vi "PID Control.vi"(8 "Reset Encoder 0":bool, 9 "M2 Setpoint":dbl(slide) scale=-0.5..0.5, 10 "M1 Setpoint":dbl(slide) scale=-0.5..0.5, 11 "M0 Setpoint":dbl(slide) scale=-1.0..1.0) -> (2 "Speed Cluster":T1, 3 "Distance Cluster":T2)   [LabVIEW 2018]
uses:
  <vilib>/addons/control/pid/pid.llb/PID (DBL).vi
  <vilib>/addons/control/pid/NI_PID_pid.lvlib
panel:
  out "dt out (s)":dbl format="%.3f"
  in  "stop":bool
  out "PID tuning Chart":dynamicdata(graph)
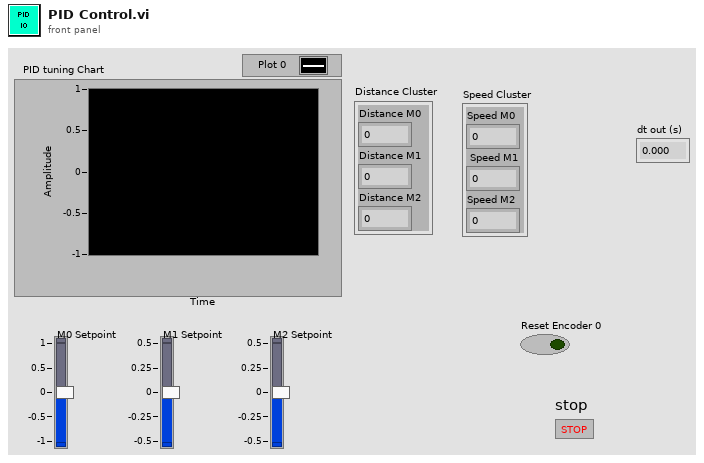
[diagram p1: front panel]
types:
  T1 = cluster{"Speed M0":dbl, " Speed M1":dbl, "Speed M2":dbl}
  T2 = cluster{"Distance M0 ":dbl, "Distance M1 ":dbl, "Distance M2 ":dbl}
  T3 = cluster{"proportional gain (Kc)":dbl, "integral time (Ti, min)":dbl, "derivative time (Td, min)":dbl}
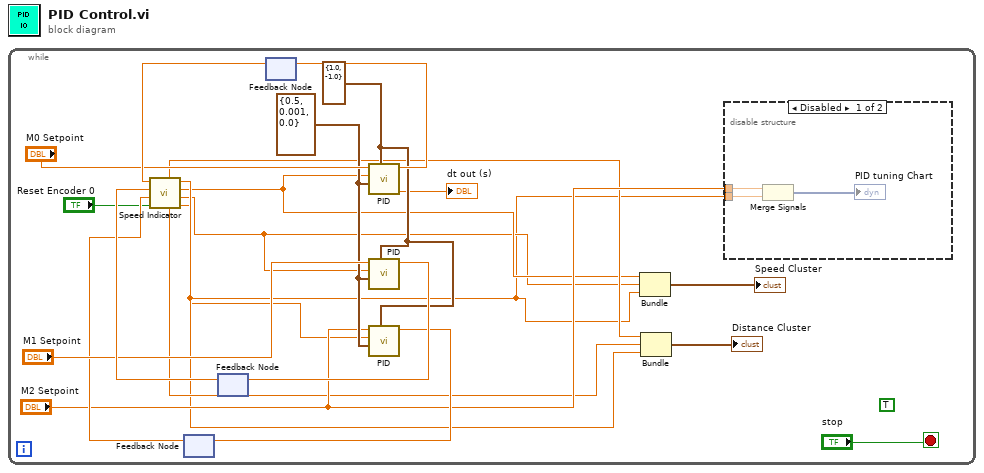
[diagram p0: block diagram]
diagram:
  n1 = while {
    stop <- "stop" stop-if-true
    (unwired) TRUE ("Boolean")
    w16 = T3 {"proportional gain (Kc)"=0.5, "integral time (Ti, min)"=0.001, "derivative time (Td, min)"=0.0} ("PID gains")
    w13 = cluster{"output high":dbl, "output low":dbl} {"output high"=1.0, "output low"=-1.0} ("output range")
    n2 = feedback #1() -> (w14:dbl)  [unwired: 1 in]
    n3 = feedback #2() -> (w18:dbl)  [unwired: 1 in]
    n4 = feedback #3() -> (w22:dbl)  [unwired: 1 in]
    n5 = call "Speed Indicator.vi"("Reset Encoder 0"="Reset Encoder 0", "Speed M2"=w14, "Speed M1 2"=w18, "Speed M0"=w22) -> ("Speed M2"=w5:dbl, "Speed M1"=w6:dbl, "Speed M0"=w7:dbl, "Distance M2"=w9:dbl, "Distance M1"=w10:dbl, "Distance M0"=w11:dbl)  [unwired: 2 in]
    n6 = call-poly <vilib>:"PID.vi"("output range"=w13, "PID gains"=w16, "process variable"=w7, "setpoint"="M0 Setpoint") -> ("dt out (s)"=→"dt out (s)":dbl, "output"=w21:dbl)  [unwired: 6 in]
    n7 = feedback-in #3(w21) -> ()
    n8 = call-poly <vilib>:"PID.vi"("output range"=w13, "PID gains"=w16, "process variable"=w6, "setpoint"="M1 Setpoint") -> ("output"=w19:dbl)  [unwired: 6 in, 1 out]
    n9 = feedback-in #2(w19) -> ()
    n10 = call-poly <vilib>:"PID.vi"("output range"=w13, "PID gains"=w16, "process variable"=w5, "setpoint"="M2 Setpoint") -> ("output"=w15:dbl)  [unwired: 6 in, 1 out]
    n11 = feedback-in #1(w15) -> ()
    n12 = Bundle("Speed M0"=w7, "Speed M1"=w6, "Speed M2"=w5) -> (→"Speed Cluster":T1)  [unwired: 1 in]
    n13 = Bundle("Distance M0"=w11, "Distance M1"=w10, "Distance M2"=w9) -> (→"Distance Cluster":T2)  [unwired: 1 in]
    n14 = disable-structure shown="Disabled" {
      disable-tunnel: "M2 Setpoint" -> [w24 _]
      disable-tunnel: w5 -> [w23 _]
      frame Disabled {
        n15 = Merge Signals(w24, w23) -> (→"PID tuning Chart":dynamicdata)
      }
      frame Enabled {
      }
    }
  }
